vi "SRX_Read Status ALL.vi"(8 "Error":errorcluster, 9 "PidLoopIdx":u32, 11 "PhoenixMotorControlDevRef":T10={"DeviceStatus"={"status"=FALSE, "code"=0, "source"=""}, "Type"=enum."PWM", "PWM"={"PWM Channel"=enum."Invalid", "DeadBand"={"Name"="", "maxPositivePwm"=0, "minPositivePwm"=0, "centerPwm"=0, "maxNegativePwm"=0, "minNegativePwm"=0, "angularRange"=0}}, "CAN"={"Device Number"=0, "SetOutput VI Ref"=variant(enum8{"Percent VBus", "Current", "Speed", "Position", "Voltage"} enum."Percent VBus"), "GetOutput VI Ref"=variant(refnum<k1> refnum), "Enable VI Ref"=variant(dbl 12.0), "Disable VI Ref"=variant(enum8{"Percent VBus", "Speed", "Position", "Slave", "Unchanged / Invalid", "Voltage Compensation", "Current", "Motion Profile"} enum."Percent VBus"), "Data"=variant}, "Invert"=FALSE, "DIO PWM"={"PWM \"Enable\" Channel"=enum."Invalid", "DIOChannel"=enum."Invalid", "PWM Rate"=0.0}}) -> (0 "Error Out":errorcluster, 1 "Analog Sensor Data Out":T8, 2 "Quad Sensor Data Out":T6, 3 "Common Runtime Data Out":T1 {"Temp" format="%.1f"; "Voltage"."Bus" format="%.3f"; "Voltage"."Output" format="%.3f"; "Voltage"."Percent" format="%.3f"; "Current" format="%.2f"}, 4 "PWM Data Out":T7, 5 "Device Info Out":T5, 6 "Hard Limits Out":T9)   [LabVIEW 2017]
uses:
  <vilib>/Rock Robotics/WPI/MotorControl/WPI_MotorControlDeviceRef.ctl
  <vilib>/Rock Robotics/WPI/MotorControl/WPI_MotorControlType.ctl
  <vilib>/Rock Robotics/SystemInterfaces/DIO/FPGA_DIOPWMChannel.ctl
  <vilib>/Rock Robotics/WPI/PWM/WPI_PWMDeadband.ctl
  <vilib>/Rock Robotics/SystemInterfaces/DIO/FPGA_DIOChannel.ctl
  TypeDefs SRX/Cluster_SRX_F and R Limit Indicators.ctl
  TypeDefs SRX/Cluster_SRX_Analog In Data.ctl
  TypeDefs SRX/Cluster_SRX_PWM Sensor Data.ctl
  TypeDefs SRX/Cluster_SRX_Sensor Quad Data.ctl
  TypeDefs SRX/Cluster_SRX_General Data.ctl
  TypeDefs SRX/Cluster_SRX_Common Runtime Data.ctl
  TypeDefs SRX/Cluster_SRX_Error Calculations.ctl
  TypeDefs SRX/Cluster_SRX_Voltage Out Data.ctl
  TypeDefs SRX/Cluster_SRX_Sensor Out Data.ctl
panel:
  # "C"
  # "Units"
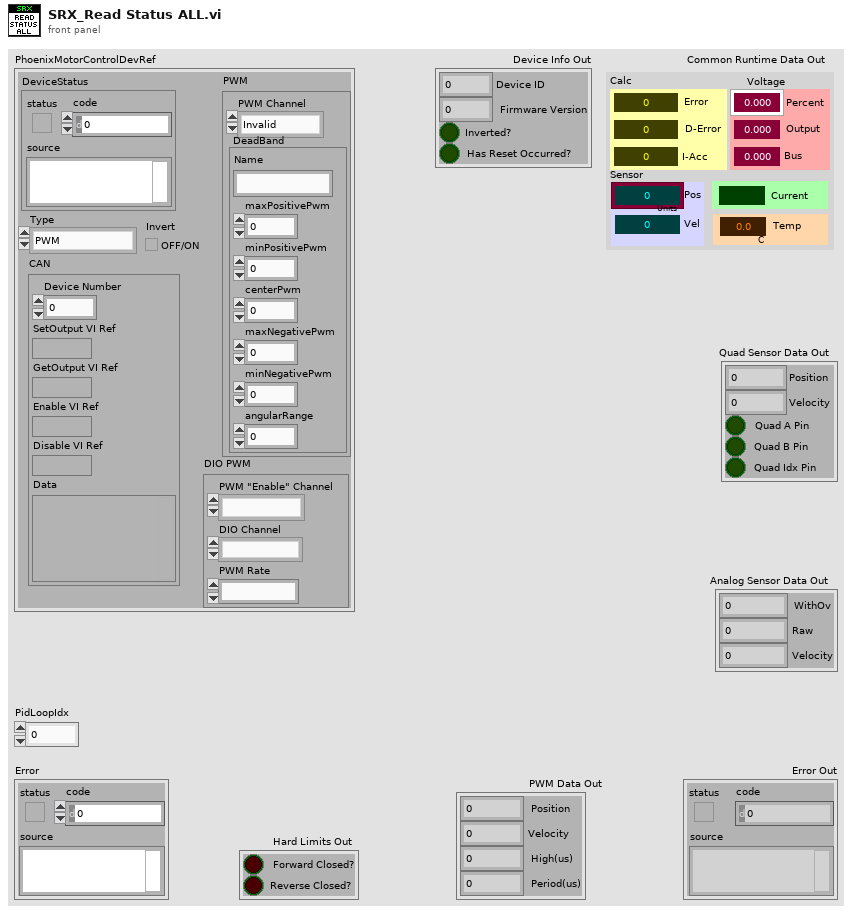
[diagram p1: front panel]
types:
  T1 = typedef "Cluster_SRX_Common Runtime Data.ctl" = cluster{"Calc":T2, "Voltage ":T3, "Sensor":T4, "Current":dbl, "Temp":dbl}
  T2 = typedef "Cluster_SRX_Error Calculations.ctl" = cluster{"Error":dbl, "D-Error":dbl, "I-Acc":dbl}
  T3 = typedef "Cluster_SRX_Voltage Out Data.ctl" = cluster{"Percent":dbl, "Output":dbl, "Bus":dbl}
  T4 = typedef "Cluster_SRX_Sensor Out Data.ctl" = cluster{"Pos":i32, "Vel":i32}
  T5 = typedef "Cluster_SRX_General Data.ctl" = cluster{"Device ID":i32, "Firmware Version":i32, "Inverted?":bool, "Has Reset Occurred?":bool}
  T6 = typedef "Cluster_SRX_Sensor Quad Data.ctl" = cluster{"Position":i32, "Velocity":i32, "Quad A Pin":bool, "Quad B Pin":bool, "Quad Idx Pin":bool}
  T7 = typedef "Cluster_SRX_PWM Sensor Data.ctl" = cluster{"Position":i32, "Velocity":i32, "High(us)":i32, "Period(us)":i32}
  T8 = typedef "Cluster_SRX_Analog In Data.ctl" = cluster{"WithOv":i32, "Raw":i32, "Velocity":i32}
  T9 = typedef "Cluster_SRX_F and R Limit Indicators.ctl" = cluster{"Forward Closed?":bool, "Reverse Closed?":bool}
  T10 = typedef "WPI_MotorControlDeviceRef.ctl" = cluster{"DeviceStatus":errorcluster, "Type":T11, "PWM":cluster{"PWM Channel":T12, "DeadBand":T13}, "CAN":cluster{"Device Number":u8, "SetOutput VI Ref":variant, "GetOutput VI Ref":variant, "Enable VI Ref":variant, "Disable VI Ref":variant, "Data":variant}, "Invert":bool, "DIO PWM":cluster{"PWM \"Enable\" Channel":T12, "DIOChannel":T14, "PWM Rate":dbl}}
  T11 = typedef "WPI_MotorControlType.ctl" = enum16{"PWM", "CAN", "DIO PWM"}
  T12 = typedef "FPGA_DIOPWMChannel.ctl" = enum8{"PWM 0", "PWM 1", "PWM 2", "PWM 3", "PWM 4", "PWM 5", "PWM 6", "PWM 7", "PWM 8", "PWM 9", "PWM MXP 0", "PWM MXP 1", "PWM MXP 2", "PWM MXP 3", "PWM MXP 4", "PWM MXP 5", "PWM MXP 6", "PWM MXP 7", "PWM MXP 8", "PWM MXP 9", "Invalid"}
  T13 = typedef "WPI_PWMDeadband.ctl" = cluster{"Name":string, "maxPositivePwm":i32, "minPositivePwm":i32, "centerPwm":i32, "maxNegativePwm":i32, "minNegativePwm":i32, "angularRange":u16}
  T14 = typedef "FPGA_DIOChannel.ctl" = enum8{"DIO 0", "DIO 1", "DIO 2", "DIO 3", "DIO 4", "DIO 5", "DIO 6", "DIO 7", "DIO 8", "DIO 9", "DIO MXP 0", "DIO MXP 1", "DIO MXP 2", "DIO MXP 3", "DIO MXP 4", "DIO MXP 5", "DIO MXP 6", "DIO MXP 7", "DIO MXP 8", "DIO MXP 9", "DIO MXP 10", "DIO MXP 11", "DIO MXP 12", "DIO MXP 13", "DIO MXP 14", "DIO MXP 15", "SPI Port CS1", "SPI Port CS2", "SPI Port CS3", "SPI Port MISO", "SPI Port MOSI", "Invalid"}
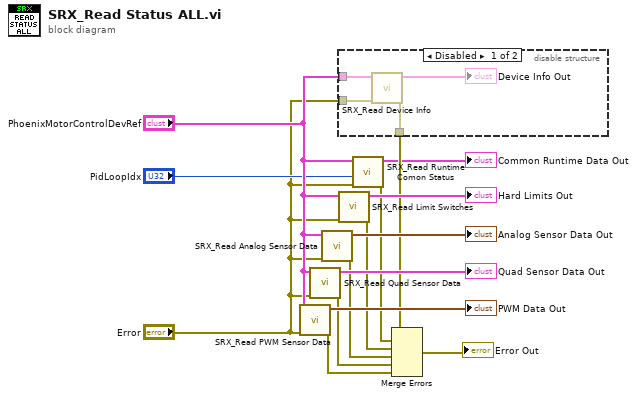
[diagram p0: block diagram]
diagram:
  n1 = call "SRX_Read PWM Sensor Data.vi"("Error"="Error", "PhoenixMotorControlDevRef"="PhoenixMotorControlDevRef") -> ("Error Out"=w8:errorcluster, "PWM Data Out"=→"PWM Data Out":T7)  [unwired: 8 in]
  n2 = call "SRX_Read Quad Sensor Data.vi"("Error"="Error", "PhoenixMotorControlDevRef"="PhoenixMotorControlDevRef") -> ("Error Out"=w9:errorcluster, "Quad Sensor Data Out"=→"Quad Sensor Data Out":T6)  [unwired: 8 in]
  n3 = call "SRX_Read Analog Sensor Data.vi"("Error"="Error", "PhoenixMotorControlDevRef"="PhoenixMotorControlDevRef") -> ("Error Out"=w10:errorcluster, "Analog Sensor Data Out"=→"Analog Sensor Data Out":T8)  [unwired: 8 in]
  n4 = disable-structure shown="Disabled" {
    disable-tunnel: [w19 _] -> w7
    disable-tunnel: "PhoenixMotorControlDevRef" -> [w18 _]
    disable-tunnel: "Error" -> [w17 _]
    frame Disabled {
      n5 = call "SRX_Read Device Info.vi"("Error"=w17, "PhoenixMotorControlDevRef"=w18) -> ("Error Out"=w19:errorcluster, "Cluster Out"=→"Device Info Out":T5)  [unwired: 8 in]
    }
    frame Enabled {
    }
  }
  n6 = call "SRX_Read Limit Switches.vi"("Error"="Error", "PhoenixMotorControlDevRef"="PhoenixMotorControlDevRef") -> ("Error Out"=w11:errorcluster, "Limits Out"=→"Hard Limits Out":T9)  [unwired: 8 in]
  n7 = call "SRX_Read Runtime Comon Status.vi"("Error"="Error", "PidLoopIdx"="PidLoopIdx", "PhoenixMotorControlDevRef"="PhoenixMotorControlDevRef") -> ("Error Out"=w6:errorcluster, "Common Runtime Data Out"=→"Common Runtime Data Out":T1)  [unwired: 7 in]
  n8 = Merge Errors(w7, w6, w11, w10, w9, w8) -> (→"Error Out":errorcluster)
